vi "axis_positions.vi"(11 "Demodulated signals":sgl[][](array[numeric])) -> (1 "Axis positions":sgl[][](array[numeric]), 2 "Differences":sgl[][](array[numeric]), 3 "Sum amplitudes":sgl[][](array[numeric]))   [LabVIEW 2013]
panel:
  # "Do basic PSD formula to extract axis positions.  These arrays are indexed by light number and then signal 0:7 (on the input) or axis 0:3  (on output)"
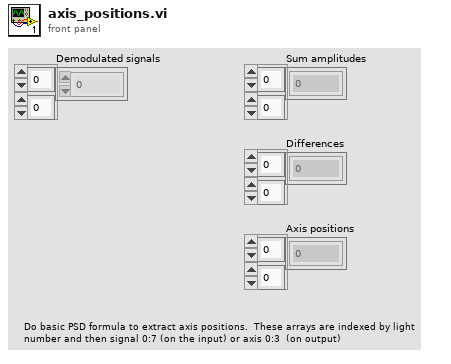
[diagram p1: front panel]
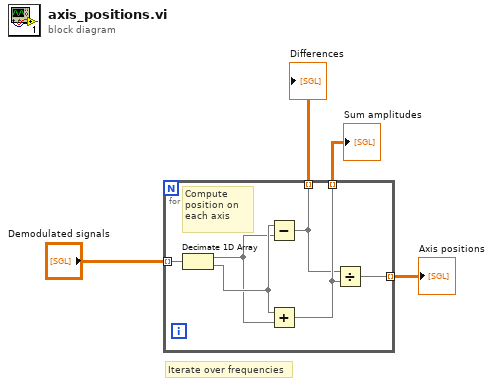
[diagram p0: block diagram]
diagram:
  # "Iterate over frequencies"
  n1 = for {
    tunnel: [w6] -> w1 mode=indexing
    tunnel: [w8] -> w4 mode=indexing
    tunnel: "Demodulated signals" -> [w7] mode=indexing
    tunnel: [w5] -> w2 mode=indexing
    # "Compute position on each axis"
    n2 = Decimate 1D Array(w7) -> (w9:sgl[], w10:sgl[])
    n3 = Subtract(x=w10, y=w9) -> (x-y=w5:sgl[])
    n4 = Add(x=w10, y=w9) -> (x+y=w6:sgl[])
    n5 = Divide(x=w5, y=w6) -> (x/y=w8:sgl[])
  }
  "Axis positions" <- w4
  "Differences" <- w2
  "Sum amplitudes" <- w1
